vi "(Depricated) AMS Gas.vi"() -> ()   [LabVIEW 2015]
uses:
  Controls/Liquid N Valve Ref Cluster.ctl
  Controls/Main Line Valve Ref Cluster.ctl
  Controls/FP Control Refs Cluster.ctl
  Controls/Sample Valve Refs.ctl
  Controls/AMS Gas State Enumerator.ctl
  Controls/Syringe Ctrl Refs.ctl
  AMS Gas/AMS Gas.lvclass
  <vilib>/ActorFramework/Stop Msg/Stop Msg.lvclass
  AMS Gas Messages/Open Thermocouples Msg/Open Thermocouples Msg.lvclass
  AMS Gas Messages/Open Log Msg/Open Log Msg.lvclass
  Controls/Sample Line State Enumerator.ctl
  AMS Gas Messages/Open Samples Msg/Open Samples Msg.lvclass
  Controls/Sample Transfer Control Enumerator.ctl
  Controls/Sample Push Control Enumerator.ctl
  Controls/Freeze Button.ctl
  Controls/Valve Custom.ctl
  Controls/Sample Transfer Container Enumerator.ctl
  Controls/Sample Transfer State Enumerator.ctl
  Controls/Sample Push State Enumerator.ctl
  Controls/Vacuum State Enumerator.ctl
panel:
  out "Sample Push Progress Slide":u8(slide) scale=0.0..100.0
  out "Sample Transfer Progress Slide":u8(slide) scale=0.0..100.0
  in  "Cylinder Home":bool
  in  "Syringe Blower":bool
  in  "Cylinder Setpoint":dbl=2.6 min=0.0 max=10.0 step=0.01 format="%_3f"
  in  "He Line Valve DV318":bool
  in  "Push Time (sec)":dbl=inf
  out "Vacuum State":T1=enum."Unknown"
  in  "Sample Push Control":T2
  in  "Sample Transfer Control":T3
  out "Sample Push State":T4
  in  "Transfer mBar":dbl min=0.0 step=1.0
  out "cRIO CPU":u8(slide) scale=0.0..100.0
  in  "Transfer Btn":bool
  in  "Target Container":T5
  in  "Source Container":T5
  out "Sample Transfer State":T6
  out "Preparation 1":bool
  out "Capillary 2":bool
  out "Capillary 1":bool
  out "Syringe pipe 1":bool
  out "Syringe pipe 2":bool
  out "Syringe pipe 3":bool
  in  "Monkey Mode":bool
  out "error out":errorcluster
  in  "FV Pump On":bool
  out "Turbo Speed":dbl format="%#_g %"
  in  "Turbo ON":bool
  in  "GV400":bool
  in  "GV401":bool
  out "FV Gauge":dbl format="%^#_3e Pa"
  in  "Open Log":bool
  out "Log":string
  in  "dvPipe 23":bool
  in  "dvPipe 21":bool
  in  "dvPipe 22":bool
  in  "dvPipe 20":bool
  in  "dvPipe 19":bool
  in  "dvPipe 18":bool
  in  "dvPipe 17":bool
  in  "dvPipe 16":bool
  in  "dvPipe 15":bool
  in  "dvPipe 14":bool
  in  "dvPipe 13":bool
  in  "dvPipe 12":bool
  in  "dvPipe 11":bool
  in  "dvPipe 10":bool
  in  "dvPipe 9":bool
  in  "dvPipe 8":bool
  in  "dvPipe 7":bool
  in  "dvPipe 6":bool
  in  "dvPipe 5":bool
  in  "dvPipe 4":bool
  in  "dvPipe 3":bool
  in  "dvPipe 2":bool
  in  "dvPipe 1":bool
  in  "VacLine 2":bool
  in  "VacLine 1":bool
  out "Syringe Position":i32(slide)
  in  "Syringe Setpoint":dbl=1.0 format="%.2f"
  in  "Syringe Enable":bool
  in  "Syringe Run":bool
  in  "Syringe Home":bool
  in  "Syringe Heater":bool
  in  "Piston Heater":bool
  in  "Syringe Freeze":bool
  in  "Syringe TC Graph":bool
  out "Syringe TC":dbl(slide) scale=-200.0..100.0
  out "Syringe Vacuum Gauge PT303":dbl(knob) scale=1.333..1333.0 scale format="%.2e"
  out "Turbo Vacuum Gauge PT302":dbl(knob) scale=1.333..1333.0 scale format="%.2e"
  in  "syrButton":bool
  in  "Liquid N Master Valve HV 107":bool
  in  "Cold Bath Syringe HV 106":bool
  in  "HV315":bool
  in  "HV314":bool
  in  "Turbo Valve DV313":bool
  out "Syringe":dbl(slide) scale=0.0..10.0
  in  "Tank Blower 4":bool
  in  "Tank Blower 3":bool
  in  "Tank Blower 2":bool
  in  "Tank Blower 1":bool
  in  "Cold Bath 1 Freeze":T7
  in  "Cold Bath 2 Freeze":T7
  in  "Cold Bath 3 Freeze":T7
  in  "Cold Bath 4 Freeze":T7
  in  "Clear Charts":bool
  in  "Cold Bath Storage 1 HV 102":T8
  in  "Cold Bath Storage 2 HV 103":T8
  in  "Cold Bath Storage 3 HV 104":bool
  in  "Cold Bath Storage 4 HV 105":bool
  out "Syringe chart":cluster{dbl, dbl}(graph)
  out "TC1":dbl(slide) scale=-200.0..30.0
  out "TC2":dbl(slide) scale=-200.0..30.0
  out "TC3":dbl(slide) scale=-200.0..30.0
  out "TC4":dbl(slide) scale=-200.0..30.0
  out "Baratrons Chart":cluster{"mean":dbl, "mean":dbl}(graph)
  out "Baratron 2":dbl(knob) scale=1.333..1333.0 scale format="%.2e"
  out "Baratron 1":dbl(knob) scale=1.333..1333.0 scale format="%.2e"
  in  "Storage Valve 1":bool
  in  "Prep Line Valve 0 DV300":bool
  in  "Storage Valve 2":bool
  in  "Storage Valve 3":bool
  in  "Storage Valve 4":bool
  in  "Storage Valve 5":bool
  in  "Storage Valve 6":bool
  in  "Storage Valve 7":bool
  in  "Storage Valve 9":bool
  in  "Storage Valve 10":bool
  in  "Storage Valve 11":bool
  in  "Storage Valve 12":bool
  in  "Sample 1 DV314":bool
  in  "Sample 2 DV315":bool
  in  "Sample 3 DV316":bool
  in  "Sample 4 DV317":bool
  in  "Sample 5 DV318":bool
  in  "Storage Valve 8":bool
  in  "Tube 1":bool
  in  "Tube 2":bool
  in  "Tube 3":bool
  in  "Tube 4":bool
  in  "Tube 5":bool
  in  "Tube 6":bool
  in  "Tube 7":bool
  in  "Tube 8":bool
  in  "Tube 9":bool
  in  "Tube 10":bool
  in  "Tube 11":bool
  in  "Tube 12":bool
  in  "Sample 1":bool
  in  "Sample 2":bool
  in  "Sample 3":bool
  in  "Sample 4":bool
  in  "Sample 5":bool
  out "Syringe":bool
  # "VS"
  # "VT"
  # "1"
  # "2"
  # "3"
  # "4"
  # "5"
  # "6"
  # "7"
  # "8"
  # "9"
  # "10"
  # "11"
  # "12"
  # "VIn"
  # "He Line"
  # "1"
  # "2"
  # "3"
  # "4"
  # "5"
  # "Scroll pump"
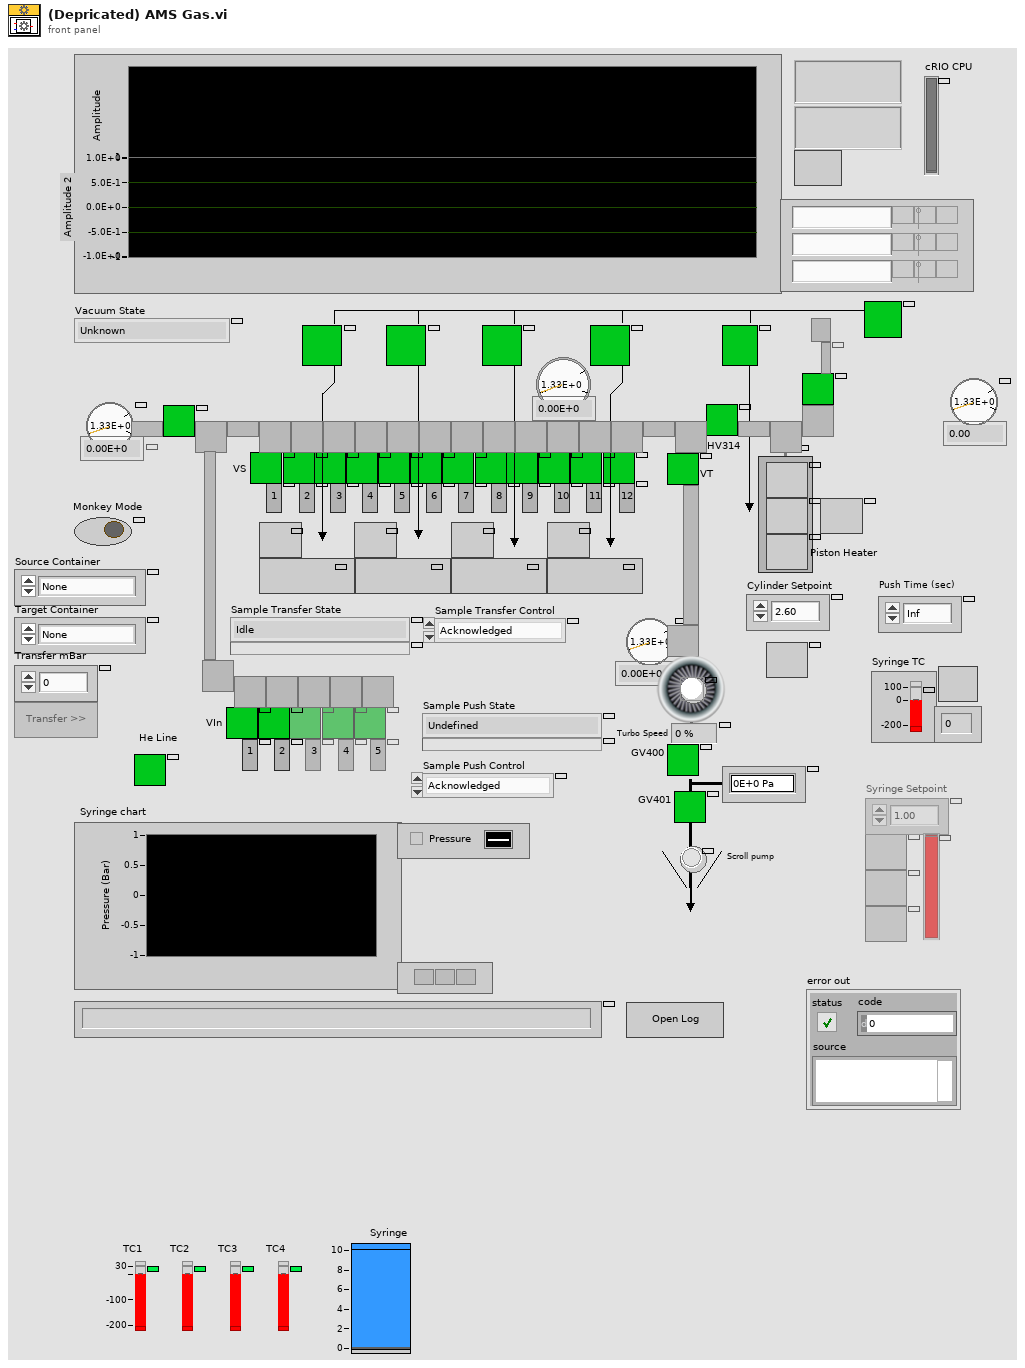
[diagram p1: front panel]
types:
  T1 = typedef "Vacuum State Enumerator.ctl" = enum16{"Pressure Rising", "Plateau", "Pressure Dropping", "Valley", "Low Valley", "Leak", "Unknown"}
  T2 = typedef "Sample Push Control Enumerator.ctl" = enum16{"Acknowledged", "Push", "Stash", "Abort", "Reset to Idle"}
  T3 = typedef "Sample Transfer Control Enumerator.ctl" = enum16{"Acknowledged", "Transfer", "Abort", "Reset to Idle"}
  T4 = typedef "Sample Push State Enumerator.ctl" = enum16{"Undefined", "Initialize", "Dilute", "Close Transfer Line", "Start Heaters", "Warm Up Syringe", "Ready to Push", "Push", "Initiate Stash", "Stash", "Complete", "Abort", "Idle", "Error"}
  T5 = typedef "Sample Transfer Container Enumerator.ctl" = enum16{"None", "Sample 1", "Sample 2", "Sample 3", "Sample 4", "Sample 5", "Storage 01", "Storage 02", "Storage 03", "Storage 04", "Storage 05", "Storage 06", "Storage 07", "Storage 08", "Storage 09", "Storage 10", "Storage 11", "Storage 12", "Syringe", "Undefined"}
  T6 = typedef "Sample Transfer State Enumerator.ctl" = enum16{"Idle", "Initialize", "Check Containers", "Check Temperatures", "Start Turbo", "Warm Up Containers", "Prepare for purging", "Purge Capillary", "Purge", "Open Containers", "Introduce Sample", "Measure Base Pressure", "Home Syringe", "Start Freezer", "Freeze Target", "Crystalize", "Stash", "Polish", "Stop Freezers", "Push Sample", "Complete", "Abort", "Error", "Undefined"}
  T7 = typedef "Freeze Button.ctl" = bool
  T8 = typedef "Valve Custom.ctl" = bool
  T9 = typedef "AMS Gas State Enumerator.ctl" = enum16{"Initialize", "Idle", "Change to Manual", "Change to Auto", "Shutdown"}
  T10 = typedef "FP Control Refs Cluster.ctl" = cluster{"Liquid N Valve References":T11, "Main Line Valve Refs":T12, "Transfer Line Container":refnum<vi>, "Storage Containers":refnum<vi>[], "Sample Refs":T13, "Syringe Ctrl Refs ":T14, "Baratrons Chart":refnum<vi>, "Capillary Container":refnum<vi>, "Preparation Container":refnum<vi>, "Monkey Mode":refnum<vi>}
  T11 = typedef "Liquid N Valve Ref Cluster.ctl" = cluster{"Cold Bath H2O HV 100":refnum<vi>, "Cold Bath Cleaning HV 101":refnum<vi>, "Cold Bath Storage 1 HV 102":refnum<vi>, "Cold Bath Storage 2 HV 103":refnum<vi>, "Cold Bath Storage 3 HV 104":refnum<vi>, "Cold Bath Storage 4 HV 105":refnum<vi>, "Cold Bath Syringe HV 106":refnum<vi>, "Liquid N Master Valve HV 107":refnum<vi>}
  T12 = typedef "Main Line Valve Ref Cluster.ctl" = cluster{"Turbo Valve DV313":refnum<vi>, "Prep Line Valve 0 DV300":refnum<vi>, "Storage Valves":refnum<vi>[]}
  T13 = typedef "Sample Valve Refs.ctl" = cluster{"Valves":cluster{"Sample 5 DV318":refnum<vi>, "Sample 4 DV317":refnum<vi>, "Sample 3 DV316":refnum<vi>, "Sample 2 DV315":refnum<vi>, "Sample 1 DV314":refnum<vi>}, "Lines":cluster{"Sample 1":refnum<vi>, "Sample 2":refnum<vi>, "Sample 3":refnum<vi>, "Sample 4":refnum<vi>, "Sample 5":refnum<vi>}}
  T14 = typedef "Syringe Ctrl Refs.ctl" = cluster{"Syringe Home":refnum<vi>, "Syringe Freeze":refnum<vi>, "Syringe TC":refnum<vi>, "Syringe Container":refnum<vi>}
  T15 = cluster{"Syringe pipe 3":refnum<vi>, "Syringe pipe 2":refnum<vi>, "Syringe pipe 1":refnum<vi>, "Syringe":refnum<vi>}
  T16 = enum8{"Enabled", "Disabled", "Disabled and Grayed Out"}
  T17 = typedef "Sample Line State Enumerator.ctl" = enum16{"All lines closed", "Sample line 1.", "Sample line 2.", "Sample line 3.", "Sample line 4.", "Sample line 5.", "Out of range"}
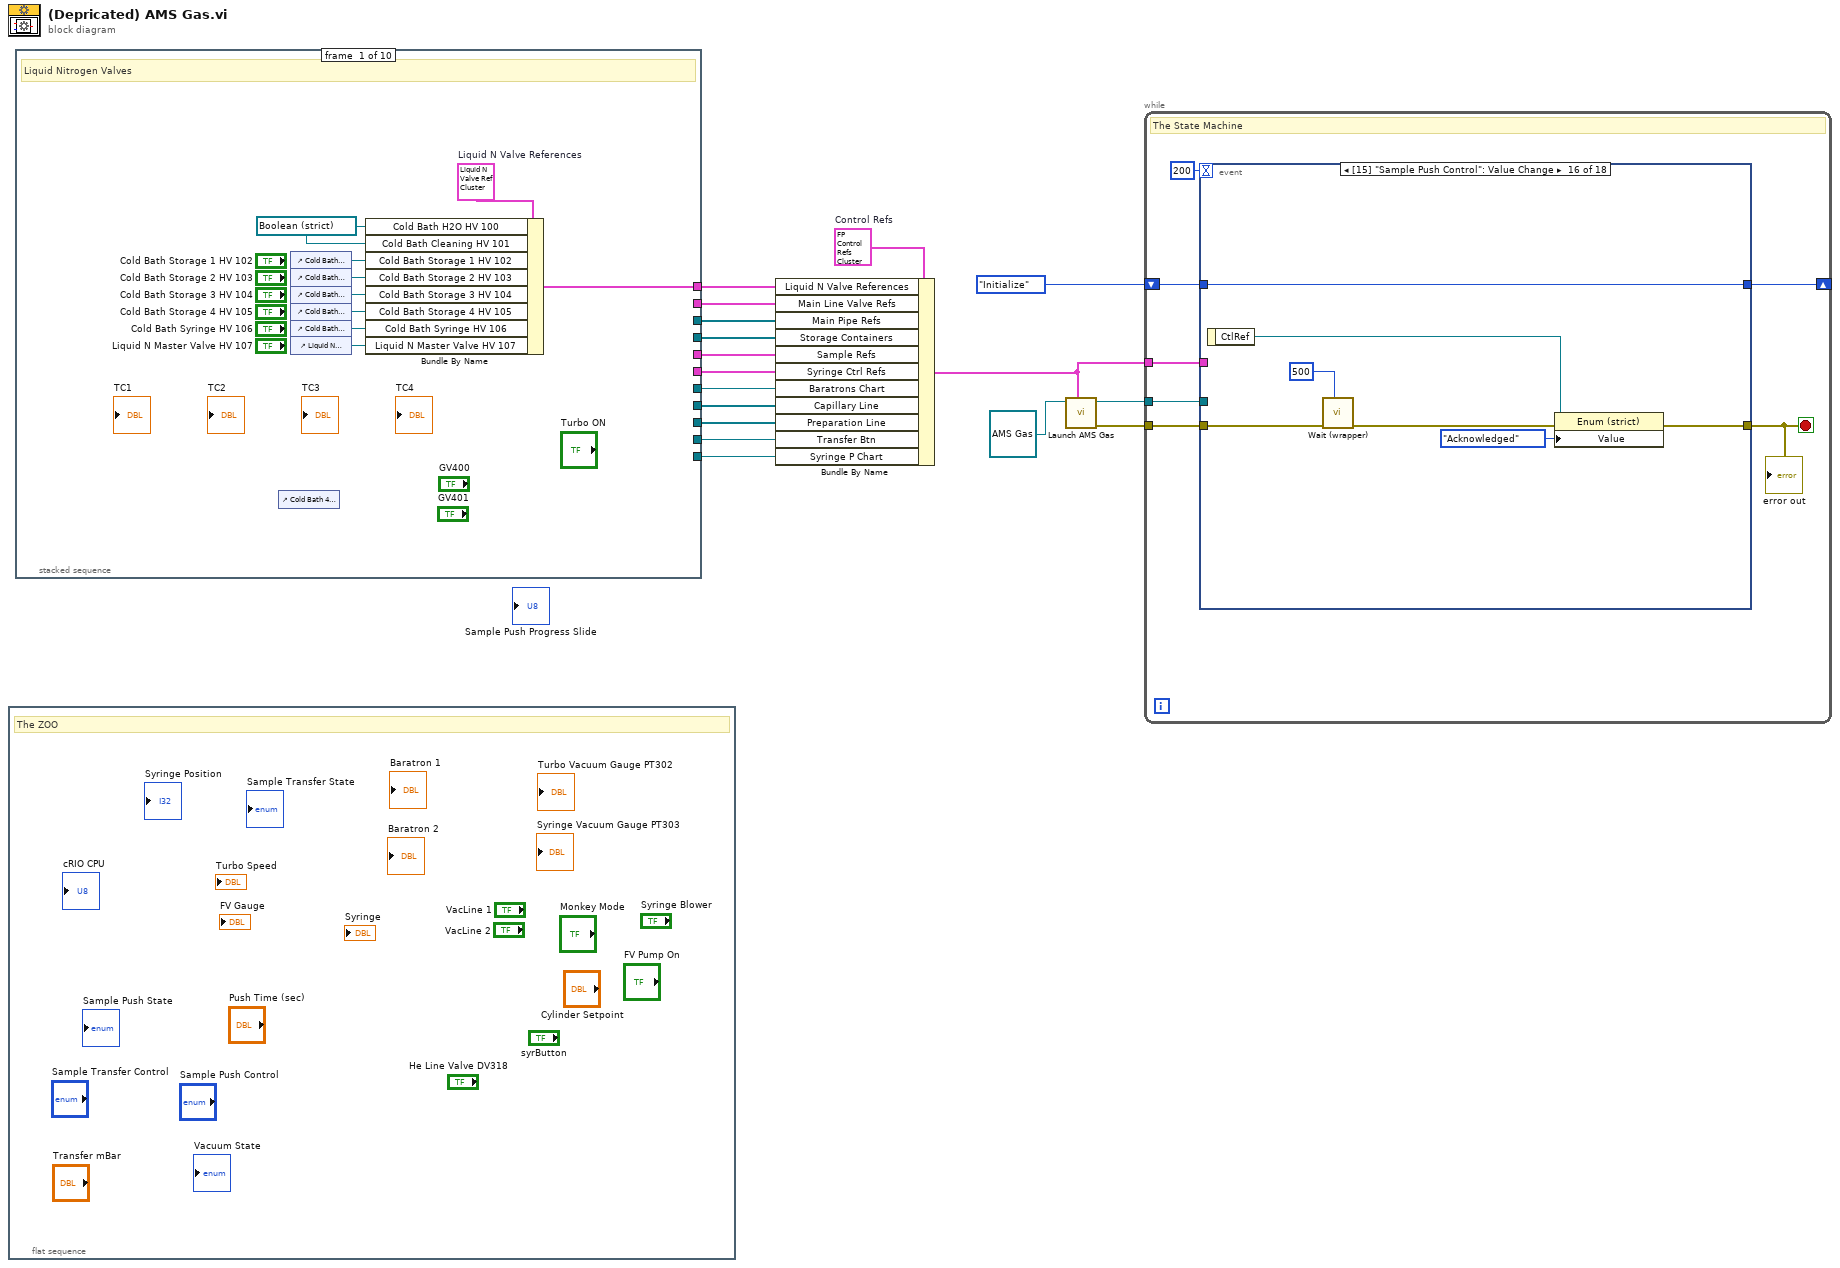
[diagram p0: block diagram]
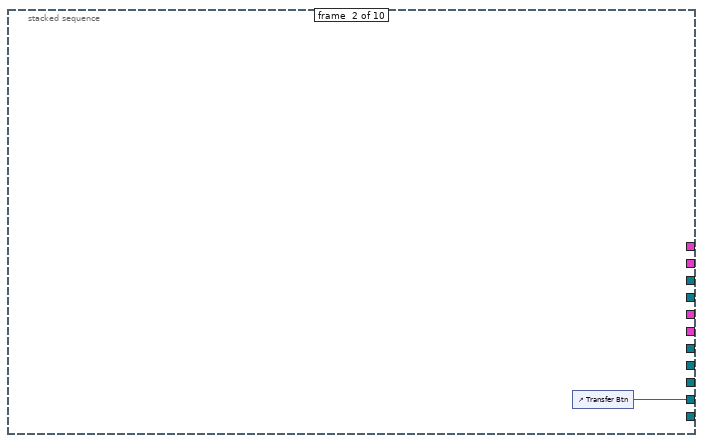
[diagram p2: hidden frame]
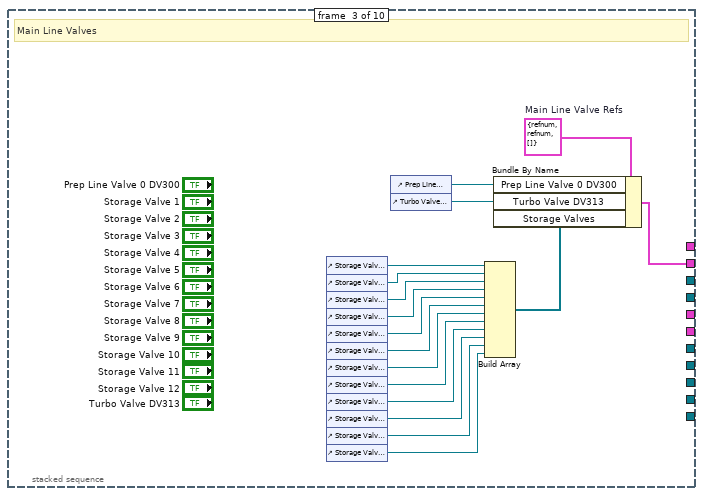
[diagram p3: hidden frame]
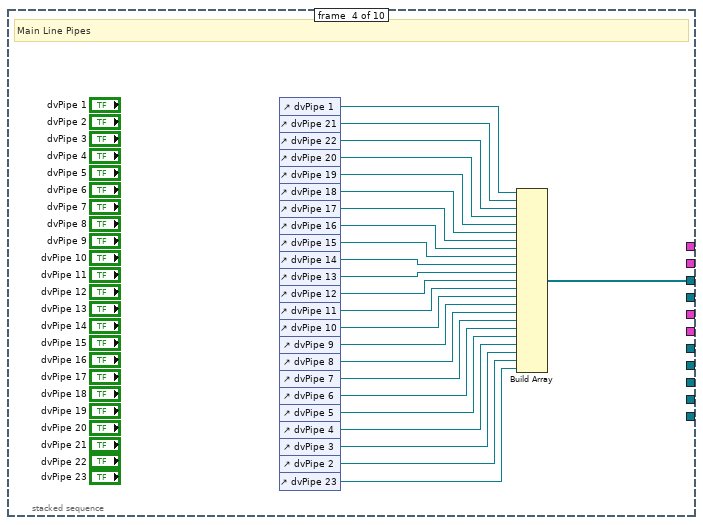
[diagram p4: hidden frame]
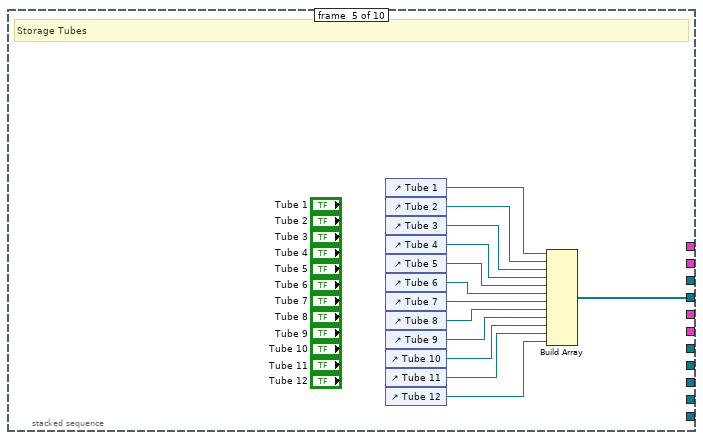
[diagram p5: hidden frame]
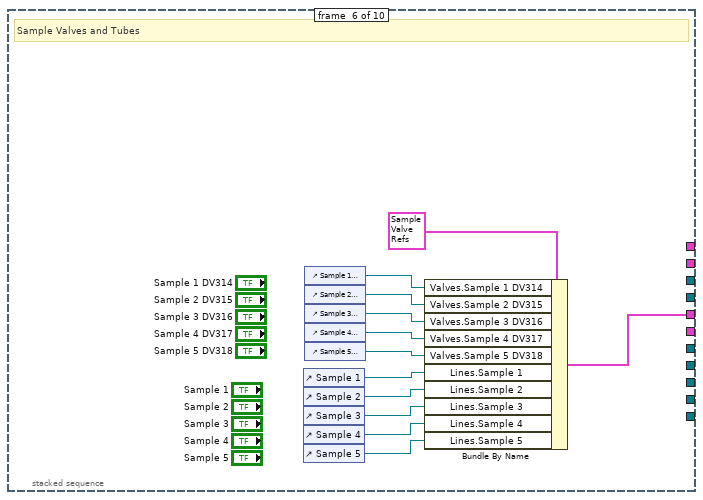
[diagram p6: hidden frame]
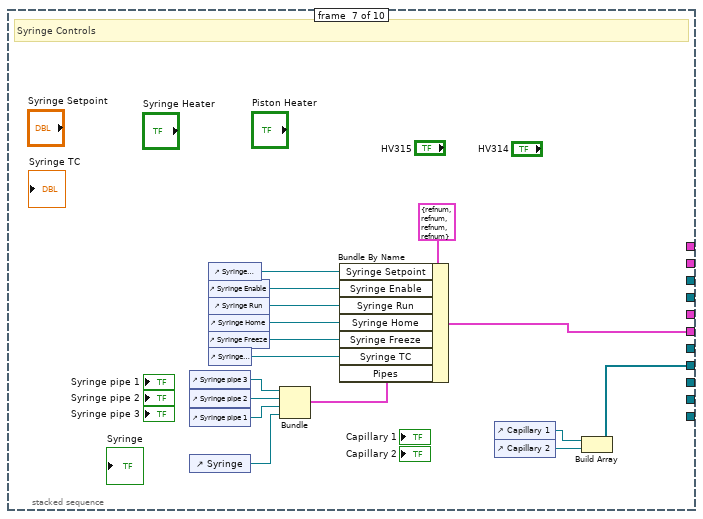
[diagram p7: hidden frame]
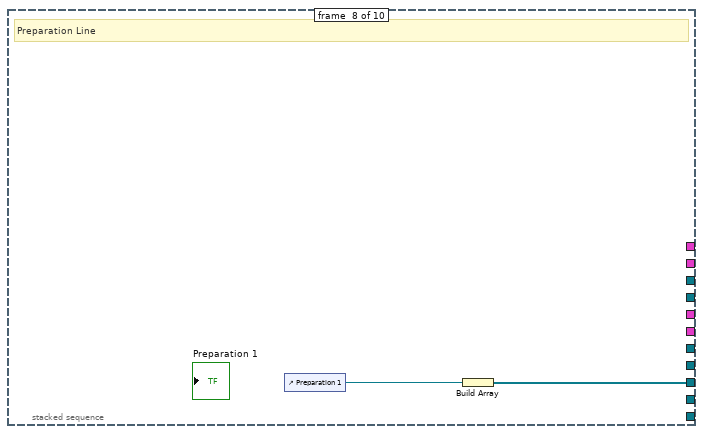
[diagram p8: hidden frame]
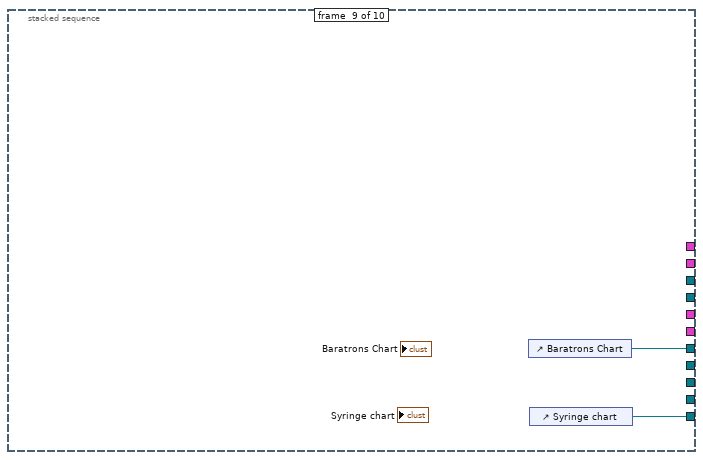
[diagram p9: hidden frame]
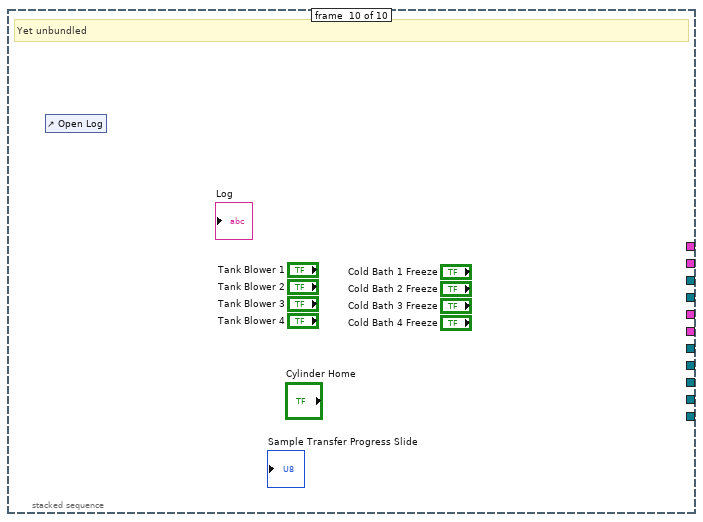
[diagram p10: hidden frame]
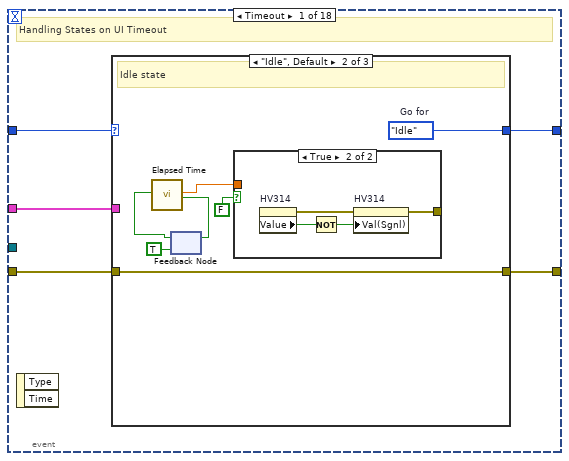
[diagram p11: hidden frame]
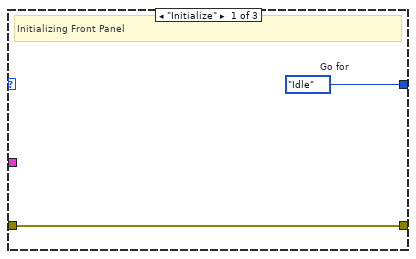
[diagram p12: hidden frame]
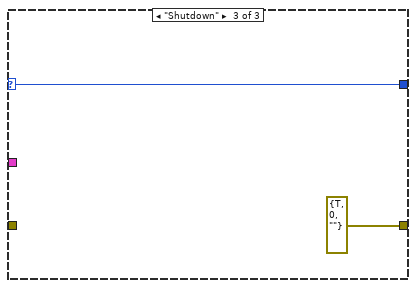
[diagram p14: hidden frame]
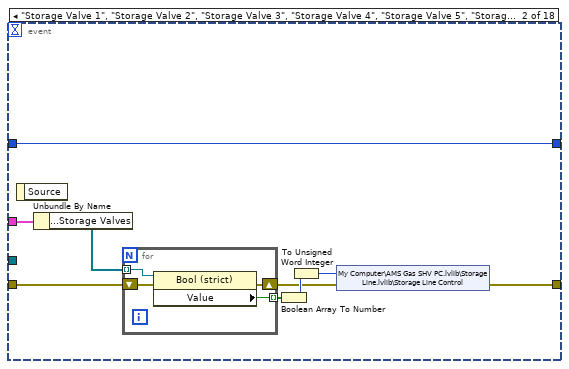
[diagram p15: hidden frame]
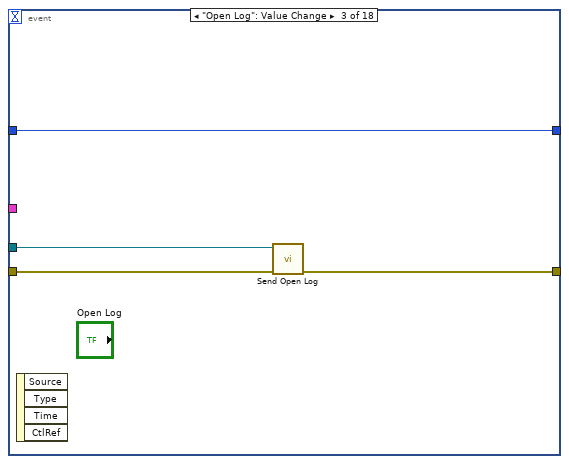
[diagram p16: hidden frame]
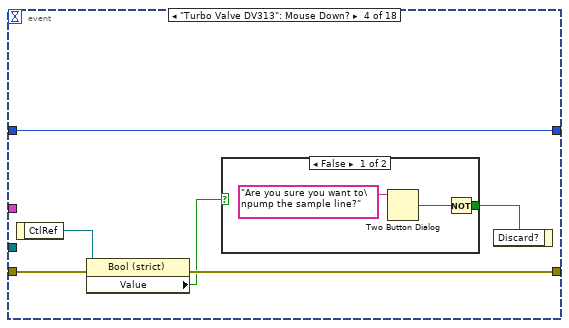
[diagram p17: hidden frame]
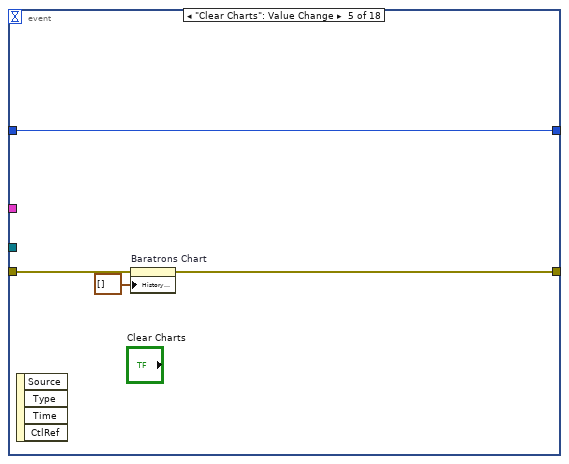
[diagram p19: hidden frame]
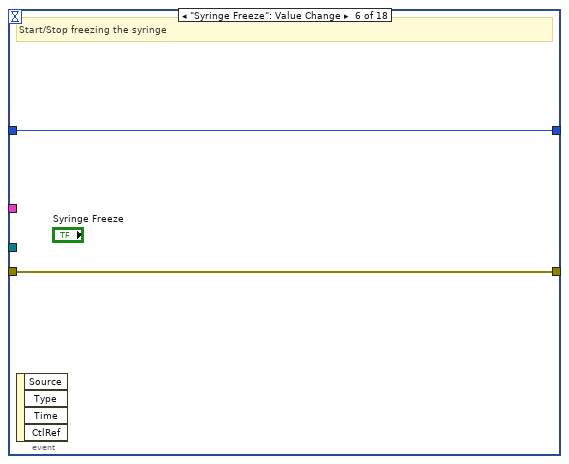
[diagram p20: hidden frame]
diagram:
  w17 = T10 {"Liquid N Valve References"={"Cold Bath H2O HV 100"=refnum, "Cold Bath Cleaning HV 101"=refnum, "Cold Bath Storage 1 HV 102"=refnum, "Cold Bath Storage 2 HV 103"=refnum, "Cold Bath Storage 3 HV 104"=refnum, "Cold Bath Storage 4 HV 105"=refnum, "Cold Bath Syringe HV 106"=refnum, "Liquid N Master Valve HV 107"=refnum}, "Main Line Valve Refs"={"Turbo Valve DV313"=refnum, "Prep Line Valve 0 DV300"=refnum, "Storage Valves"=[]}, "Transfer Line Container"=refnum, "Storage Containers"=[], "Sample Refs"={"Valves"={"Sample 5 DV318"=refnum, "Sample 4 DV317"=refnum, "Sample 3 DV316"=refnum, "Sample 2 DV315"=refnum, "Sample 1 DV314"=refnum}, "Lines"={"Sample 1"=refnum, "Sample 2"=refnum, "Sample 3"=refnum, "Sample 4"=refnum, "Sample 5"=refnum}}, "Syringe Ctrl Refs "={"Syringe Home"=refnum, "Syringe Freeze"=refnum, "Syringe TC"=refnum, "Syringe Container"=refnum}, "Baratrons Chart"=refnum, "Capillary Container"=refnum, "Preparation Container"=refnum, "Monkey Mode"=refnum}  # Control Refs
  n1 = flat-sequence {
    frame #0 {
      # "The ZOO"
    }
  }
  n2 = stacked-sequence {
    tunnel: [_ _ w44 _ _ _ _ _ _ _] -> w16
    tunnel: [_ _ _ w46 _ _ _ _ _ _] -> w14
    tunnel: [_ _ _ _ w69 _ _ _ _ _] -> w12
    tunnel: [_ _ _ _ _ w87 _ _ _ _] -> w11
    tunnel: [w19 _ _ _ _ _ _ _ _ _] -> w13
    tunnel: [_ _ _ _ _ _ w105 _ _ _] -> w10
    tunnel: [_ _ _ _ _ _ _ _ w113 _] -> w7
    tunnel: [_ _ _ _ _ _ w94 _ _ _] -> w5
    tunnel: [_ _ _ _ _ _ _ w110 _ _] -> w4
    tunnel: [_ w27 _ _ _ _ _ _ _ _] -> w3
    tunnel: [_ _ _ _ _ _ _ _ w112 _] -> w1
    frame #0 {
      w18 = refnum<vi> refnum ("Cold Bath H2O HV 100")
      w26 = T11 {"Cold Bath H2O HV 100"=refnum, "Cold Bath Cleaning HV 101"=refnum, "Cold Bath Storage 1 HV 102"=refnum, "Cold Bath Storage 2 HV 103"=refnum, "Cold Bath Storage 3 HV 104"=refnum, "Cold Bath Storage 4 HV 105"=refnum, "Cold Bath Syringe HV 106"=refnum, "Liquid N Master Valve HV 107"=refnum}  # Liquid N Valve References
      # "Liquid Nitrogen Valves"
      n3 = control-ref of="Cold Bath 4 Freeze"() -> ()  [unwired: 1 out]
      n4 = control-ref of="Cold Bath Storage 1 HV 102"() -> (w20:refnum<vi>)
      n5 = control-ref of="Cold Bath Storage 2 HV 103"() -> (w21:refnum<vi>)
      n6 = control-ref of="Cold Bath Storage 3 HV 104"() -> (w22:refnum<vi>)
      n7 = control-ref of="Cold Bath Storage 4 HV 105"() -> (w23:refnum<vi>)
      n8 = control-ref of="Cold Bath Syringe HV 106"() -> (w24:refnum<vi>)
      n9 = control-ref of="Liquid N Master Valve HV 107"() -> (w25:refnum<vi>)
      n10 = Bundle By Name(cluster=w26, "Cold Bath H2O HV 100"=w18, "Cold Bath Cleaning HV 101"=w18, "Cold Bath Storage 1 HV 102"=w20, "Cold Bath Storage 2 HV 103"=w21, "Cold Bath Storage 3 HV 104"=w22, "Cold Bath Storage 4 HV 105"=w23, "Cold Bath Syringe HV 106"=w24, "Liquid N Master Valve HV 107"=w25) -> (w19:T11)
    }
    frame #1 {
      n11 = control-ref of="Transfer Btn"() -> (w27:refnum<vi>)
    }
    frame #2 {
      w42 = T12 {"Turbo Valve DV313"=refnum, "Prep Line Valve 0 DV300"=refnum, "Storage Valves"=[]}  # Main Line Valve Refs
      # "Main Line Valves"
      n12 = control-ref of="Storage Valve 1"() -> (w40:refnum<vi>)
      n13 = control-ref of="Storage Valve 2"() -> (w39:refnum<vi>)
      n14 = control-ref of="Storage Valve 3"() -> (w38:refnum<vi>)
      n15 = control-ref of="Storage Valve 4"() -> (w37:refnum<vi>)
      n16 = control-ref of="Storage Valve 5"() -> (w36:refnum<vi>)
      n17 = control-ref of="Storage Valve 6"() -> (w35:refnum<vi>)
      n18 = control-ref of="Storage Valve 7"() -> (w34:refnum<vi>)
      n19 = control-ref of="Storage Valve 8"() -> (w33:refnum<vi>)
      n20 = control-ref of="Storage Valve 9"() -> (w32:refnum<vi>)
      n21 = control-ref of="Storage Valve 10"() -> (w31:refnum<vi>)
      n22 = control-ref of="Storage Valve 11"() -> (w30:refnum<vi>)
      n23 = control-ref of="Storage Valve 12"() -> (w29:refnum<vi>)
      n24 = control-ref of="Prep Line Valve 0 DV300"() -> (w43:refnum<vi>)
      n25 = control-ref of="Turbo Valve DV313"() -> (w41:refnum<vi>)
      n26 = Build Array(w40, w39, w38, w37, w36, w35, w34, w33, w32, w31, w30, w29) -> (w28:refnum<vi>[])
      n27 = Bundle By Name(cluster=w42, "Prep Line Valve 0 DV300"=w43, "Turbo Valve DV313"=w41, "Storage Valves"=w28) -> (w44:T12)
    }
    frame #3 {
      # "Main Line Pipes"
      n28 = control-ref of="dvPipe 1"() -> (w47:refnum<vi>)
      n29 = control-ref of="dvPipe 21"() -> (w48:refnum<vi>)
      n30 = control-ref of="dvPipe 22"() -> (w49:refnum<vi>)
      n31 = control-ref of="dvPipe 20"() -> (w50:refnum<vi>)
      n32 = control-ref of="dvPipe 19"() -> (w51:refnum<vi>)
      n33 = control-ref of="dvPipe 18"() -> (w52:refnum<vi>)
      n34 = control-ref of="dvPipe 17"() -> (w53:refnum<vi>)
      n35 = control-ref of="dvPipe 16"() -> (w54:refnum<vi>)
      n36 = control-ref of="dvPipe 15"() -> (w55:refnum<vi>)
      n37 = control-ref of="dvPipe 14"() -> (w56:refnum<vi>)
      n38 = control-ref of="dvPipe 13"() -> (w57:refnum<vi>)
      n39 = control-ref of="dvPipe 12"() -> (w58:refnum<vi>)
      n40 = control-ref of="dvPipe 11"() -> (w59:refnum<vi>)
      n41 = control-ref of="dvPipe 10"() -> (w60:refnum<vi>)
      n42 = control-ref of="dvPipe 9"() -> (w61:refnum<vi>)
      n43 = control-ref of="dvPipe 8"() -> (w62:refnum<vi>)
      n44 = control-ref of="dvPipe 7"() -> (w63:refnum<vi>)
      n45 = control-ref of="dvPipe 6"() -> (w64:refnum<vi>)
      n46 = control-ref of="dvPipe 5"() -> (w65:refnum<vi>)
      n47 = control-ref of="dvPipe 4"() -> (w66:refnum<vi>)
      n48 = control-ref of="dvPipe 3"() -> (w67:refnum<vi>)
      n49 = control-ref of="dvPipe 2"() -> (w68:refnum<vi>)
      n50 = control-ref of="dvPipe 23"() -> (w45:refnum<vi>)
      n51 = Build Array(w47, w48, w49, w50, w51, w52, w53, w54, w55, w56, w57, w58, w59, w60, w61, w62, w63, w64, w65, w66, w67, w68, w45) -> (w46:refnum<vi>[])
    }
    frame #4 {
      # "Storage Tubes"
      n52 = control-ref of="Tube 1"() -> (w74:refnum<vi>)
      n53 = control-ref of="Tube 2"() -> (w75:refnum<vi>)
      n54 = control-ref of="Tube 3"() -> (w78:refnum<vi>)
      n55 = control-ref of="Tube 4"() -> (w77:refnum<vi>)
      n56 = control-ref of="Tube 5"() -> (w76:refnum<vi>)
      n57 = control-ref of="Tube 6"() -> (w72:refnum<vi>)
      n58 = control-ref of="Tube 7"() -> (w79:refnum<vi>)
      n59 = control-ref of="Tube 8"() -> (w71:refnum<vi>)
      n60 = control-ref of="Tube 9"() -> (w73:refnum<vi>)
      n61 = control-ref of="Tube 10"() -> (w80:refnum<vi>)
      n62 = control-ref of="Tube 11"() -> (w81:refnum<vi>)
      n63 = control-ref of="Tube 12"() -> (w70:refnum<vi>)
      n64 = Build Array(w74, w75, w78, w77, w76, w72, w79, w71, w73, w80, w81, w70) -> (w69:refnum<vi>[])
    }
    frame #5 {
      # "Sample Valves and Tubes"
      n65 = control-ref of="Sample 1"() -> (w86:refnum<vi>)
      n66 = control-ref of="Sample 2"() -> (w85:refnum<vi>)
      n67 = control-ref of="Sample 3"() -> (w84:refnum<vi>)
      n68 = control-ref of="Sample 4"() -> (w83:refnum<vi>)
      n69 = control-ref of="Sample 5"() -> (w82:refnum<vi>)
      n70 = control-ref of="Sample 1 DV314"() -> (w93:refnum<vi>)
      n71 = control-ref of="Sample 2 DV315"() -> (w92:refnum<vi>)
      n72 = control-ref of="Sample 3 DV316"() -> (w91:refnum<vi>)
      n73 = control-ref of="Sample 4 DV317"() -> (w90:refnum<vi>)
      n74 = control-ref of="Sample 5 DV318"() -> (w89:refnum<vi>)
      n75 = Bundle By Name(cluster=T13 {"Valves"={"Sample 5 DV318"=refnum, "Sample 4 DV317"=refnum, "Sample 3 DV316"=refnum, "Sample 2 DV315"=refnum, "Sample 1 DV314"=refnum}, "Lines"={"Sample 1"=refnum, "Sample 2"=refnum, "Sample 3"=refnum, "Sample 4"=refnum, "Sample 5"=refnum}} ("Sample Valve Refs"), "Valves.Sample 1 DV314"=w93, "Valves.Sample 2 DV315"=w92, "Valves.Sample 3 DV316"=w91, "Valves.Sample 4 DV317"=w90, "Valves.Sample 5 DV318"=w89, "Lines.Sample 1"=w86, "Lines.Sample 2"=w85, "Lines.Sample 3"=w84, "Lines.Sample 4"=w83, "Lines.Sample 5"=w82) -> (w87:T13)
    }
    frame #6 {
      # "Syringe Controls"
      n76 = control-ref of="Syringe pipe 3"() -> (w101:refnum<vi>)
      n77 = control-ref of="Syringe pipe 2"() -> (w100:refnum<vi>)
      n78 = control-ref of="Syringe pipe 1"() -> (w99:refnum<vi>)
      n79 = control-ref of="Syringe"() -> (w97:refnum<vi>)
      n80 = control-ref of="Syringe Setpoint"() -> (w109:refnum<vi>)
      n81 = control-ref of="Syringe Enable"() -> (w108:refnum<vi>)
      n82 = control-ref of="Syringe Run"() -> (w107:refnum<vi>)
      n83 = control-ref of="Syringe Home"() -> (w104:refnum<vi>)
      n84 = control-ref of="Syringe Freeze"() -> (w103:refnum<vi>)
      n85 = control-ref of="Syringe TC"() -> (w102:refnum<vi>)
      n86 = Bundle("Syringe pipe 3"=w101, "Syringe pipe 2"=w100, "Syringe pipe 1"=w99, "Syringe"=w97) -> (w98:T15)  [unwired: 1 in]
      n87 = Bundle By Name(cluster=T14 {"Syringe Home"=refnum, "Syringe Freeze"=refnum, "Syringe TC"=refnum, "Syringe Container"=refnum} ("Syringe Ctrl Refs"), "Syringe Setpoint"=w109, "Syringe Enable"=w108, "Syringe Run"=w107, "Syringe Home"=w104, "Syringe Freeze"=w103, "Syringe TC"=w102, "Pipes"=w98) -> (w105:T14)
      n88 = control-ref of="Capillary 1"() -> (w95:refnum<vi>)
      n89 = control-ref of="Capillary 2"() -> (w96:refnum<vi>)
      n90 = Build Array(w95, w96) -> (w94:refnum<vi>[])
    }
    frame #7 {
      # "Preparation Line"
      n91 = control-ref of="Preparation 1"() -> (w111:refnum<vi>)
      n92 = Build Array(w111) -> (w110:refnum<vi>[])
    }
    frame #8 {
      n93 = control-ref of="Baratrons Chart"() -> (w113:refnum<vi>)
      n94 = control-ref of="Syringe chart"() -> (w112:refnum<vi>)
    }
    frame #9 {
      # "Yet unbundled"
      n95 = control-ref of="Open Log"() -> ()  [unwired: 1 out]
    }
  }
  n96 = Bundle By Name(cluster=w17, "Liquid N Valve References"=w13, "Main Line Valve Refs"=w16, "Main Pipe Refs"=w14, "Storage Containers"=w12, "Sample Refs"=w11, "Syringe Ctrl Refs"=w10, "Baratrons Chart"=w7, "Capillary Line"=w5, "Preparation Line"=w4, "Transfer Btn"=w3, "Syringe P Chart"=w1) -> (w2:T10)
  n97 = call "Launch AMS Gas.vi"("Control Refs"=w2, "AMS Gas in"=refnum<class "AMS Gas.lvclass"> refnum) -> ("error out"=w6:errorcluster, "Caller-To-Actor Enqueuer"=w9:refnum<class "Message Enqueuer.lvclass">)  [unwired: 7 in, 1 out]
  n98 = while {
    tunnel: w2 -> [w115]
    tunnel: w6 -> [w120]
    shift-right: [w116] -> _
    shift-left: AMS_Gas_State_Enumerator."Initialize" ("Go for") -> [w117]
    tunnel: w9 -> [w114]
    stop <- w119 stop-if-true
    # "The State Machine"
    n99 = event shown="[15] \"Sample Push Control\": Value Change" {
      selector: _ -> [_ _ _ _ _ _ _ _ _ _ _ _ _ _ _ _ _ _]
      dyn-events: _ -> [_ _ _ _ _ _ _ _ _ _ _ _ _ _ _ _ _ _]
      timeout: 200 -> [_ _ _ _ _ _ _ _ _ _ _ _ _ _ _ _ _ _]
      tunnel: w120 -> [w125 w147 w156 w161 w170 w171 w173 w177 w181 w195 w199 w233 w244 w246 w253 w295 w303 w314]
      tunnel: [w124 w142 w155 w160 w167 w171 w173 w175 w180 w191 w197 w223 w243 w246 w252 w296 w302 w313] -> w119
      tunnel: w117 -> [w123 w149 w157 w163 w169 w172 w174 w178 _ w187 w202 w234 w245 w247 w256 w299 w301 w312]
      tunnel: [w122 w149 w157 w163 w169 w172 w174 w178 w183 w187 w202 w234 w245 w247 w256 w299 w301 w312] -> w116
      tunnel: w115 -> [w121 w148 _ _ _ _ _ _ _ w196 _ _ _ _ _ _ w304 w315]
      tunnel: w114 -> [_ _ w154 _ _ _ _ w176 w179 _ w201 _ _ _ _ _ _ _]
      event Timeout {
        # "Handling States on UI Timeout"
        n100 = event-data() -> ()  [unwired: 1 in, 2 out]
        n101 = case shown="\"Idle\", Default" w123 {
          selector: w123 -> [_ _ w140]
          tunnel: w125 -> [w126 w133 _]
          tunnel: [w126 w133 errorcluster {"status"=TRUE, "code"=0, "source"=""} ("no error")] -> w124
          tunnel: [w127 w134 w140] -> w122
          tunnel: w121 -> [_ _ _]
          frame "Initialize" {
            w127 = AMS_Gas_State_Enumerator."Idle"  # Go for
            # "Initializing Front Panel"
          }
          frame "Idle", Default {
            w134 = AMS_Gas_State_Enumerator."Idle"  # Go for
            # "Idle state"
            n102 = feedback #1(TRUE ("Time has Elapsed")) -> (w132:bool)
            n103 = call "Elapsed Time"("Reset"=w132) -> ("Elapsed Time (s)"=w130:dbl, "Time has Elapsed"=w129:bool)  [unwired: 11 in, 6 out]
            n104 = feedback-in #1(w129) -> ()
            n105 = case shown="True" FALSE {
              tunnel: [_ w135] -> _
              tunnel: w130 -> [_ _]
              frame False {
              }
              frame True {
                n106 = property on="HV314" class="Bool (strict)"() -> (error out=w136:errorcluster, "Value"=w138:bool)  [unwired: 2 in, 1 out]
                n107 = Not(x=w138) -> (.not. x?=w137:bool)
                n108 = property on="HV314" class="Bool (strict)"(error in=w136, "Val(Sgnl)"=w137) -> (error out=w135:errorcluster)  [unwired: 1 in, 1 out]
              }
            }
          }
          frame "Shutdown" {
          }
        }
      }
      event "Storage Valve 1", "Storage Valve 2", "Storage Valve 3", "Storage Valve 4", "Storage Valve 5", "Storage Valve 6", "Storage Valve 7", "Storage Valve 9", "Storage Valve 10", "Storage Valve 11", "Storage Valve 12", "Storage Valve 8": Value Change {
        n109 = event-data() -> ()  [unwired: 1 in, 1 out]
        n110 = Unbundle By Name(w148) -> ("Main Line Valve Refs.Storage Valves"=w141:refnum<vi>[])
        n111 = for {
          tunnel: w141 -> [w151] mode=indexing
          tunnel: [w150] -> w146 mode=indexing
          shift-right: [w152] -> w144
          shift-left: w147 -> [w153]
          n112 = property class="Bool (strict)"(reference=w151, error in=w153) -> (error out=w152:errorcluster, "Value"=w150:bool)  [unwired: 1 out]
        }
        n113 = Boolean Array To Number(Boolean array=w146) -> (number=w145:u32)
        n114 = To Unsigned Word Integer(number=w145) -> (unsigned 16bit integer=w143:u16)
        n115 = shared-variable "My Computer\\AMS Gas SHV PC.lvlib\\Storage Line.lvlib\\Storage Line Control"(w143, error in=w144) -> (error out=w142:errorcluster)
      }
      event "Open Log": Value Change {
        n116 = event-data() -> ()  [unwired: 1 in, 4 out]
        n117 = call "Send Open Log.vi"("error in (no error)"=w156, "Message Enqueuer"=w154) -> ("error out"=w155:errorcluster)  [unwired: 8 in, 1 out]
      }
      event "Turbo Valve DV313": Mouse Down? {
        n118 = event-data() -> ("CtlRef"=w159:refnum<vi>)  [unwired: 1 in]
        n119 = property class="Bool (strict)"(reference=w159, error in=w161) -> (error out=w160:errorcluster, "Value"=w158:bool)  [unwired: 1 out]
        n120 = case shown="False" w158 {
          tunnel: [w165 _] -> w162
          frame False {
            n121 = Two Button Dialog(message="Are you sure you want to\npump the sample line?") -> (T button?=w166:bool)  [unwired: 2 in]
            n122 = Not(x=w166) -> (.not. x?=w165:bool)
          }
          frame True {
          }
        }
        n123 = event-data("Discard?"=w162) -> ()  [unwired: 1 in, 1 out]
      }
      event "Clear Charts": Value Change {
        n124 = event-data() -> ()  [unwired: 1 in, 4 out]
        n125 = property on="Baratrons Chart" class="WFChart (strict)"(error in=w170, "History Data"=cluster{"mean":dbl, "mean":dbl}[] []) -> (error out=w167:errorcluster)  [unwired: 1 in, 1 out]
      }
      event "Syringe Freeze": Value Change {
        # "Start/Stop freezing the syringe"
        n126 = event-data() -> ()  [unwired: 1 in, 4 out]
      }
      event Value Change {
        # "Start/Stop freezing the Cold Bath 4"
        n127 = event-data() -> ()  [unwired: 1 in, 4 out]
      }
      event "Syringe TC Graph": Value Change {
        n128 = event-data() -> ()  [unwired: 1 in, 4 out]
        n129 = call "Send Open Thermocouples.vi"("error in (no error)"=w177, "Message Enqueuer"=w176) -> ("error out"=w175:errorcluster)  [unwired: 8 in, 1 out]
      }
      event Panel Close? {
        w183 = AMS_Gas_State_Enumerator."Shutdown"  # Go for
        # "User closes Front Panel"
        n130 = event-data() -> ()  [unwired: 1 in, 3 out]
        n131 = call <vilib>:"Send Normal Stop.vi"("error in (no error)"=w181, "Message Enqueuer"=w179) -> ("error out"=w180:errorcluster)  [unwired: 9 in]
        n132 = event-data("Discard?"=TRUE) -> ()  [unwired: 1 in, 1 out]
      }
      event "Syringe Enable": Value Change {
        n133 = event-data() -> ()  [unwired: 1 in, 4 out]
        n134 = Unbundle By Name(w196) -> ("Syringe Run"=w192:refnum<vi>, "Syringe Ctrl Refs.Syringe Home"=w193:refnum<vi>)
        n135 = Select(t=T16."Enabled" ("Disabled"), s="Syringe Enable", f=T16."Disabled and Grayed Out" ("Disabled")) -> (s? t:f=w186:T16)
        n136 = property class="Bool (strict)"(reference=w193, error in=w195, "Value"=FALSE, "DisabledEnum"=w186) -> (error out=w194:errorcluster)  [unwired: 1 out]
        n137 = property class="Bool (strict)"(reference=w192, error in=w194, "Value"=FALSE, "DisabledEnum"=w186) -> (error out=w191:errorcluster)  [unwired: 1 out]
      }
      event "Sample 1", "Sample 2", "Sample 3", "Sample 4", "Sample 5": Mouse Down? {
        n138 = event-data() -> ("CtlRef"=w198:refnum<vi>)  [unwired: 1 in]
        n139 = disable-structure shown="Disabled" {
          disable-tunnel: w201 -> [w211 w220]
          disable-tunnel: w199 -> [w210 w222]
          disable-tunnel: w198 -> [w208 _]
          disable-tunnel: [w205 w221] -> w197
          frame Disabled {
            n140 = property class="Bool (strict)"(reference=w208, error in=w210) -> (reference out=w203:refnum<vi>, error out=w209:errorcluster, "Label.Text"=w204:string)
            n141 = call "(Depricated) Dialog Sample.vi"("Sample Line Control Ref"=w203, "Error In"=w209, "Caller-To-Actor Enqueuer"=w211) -> ("Error Out"=w207:errorcluster, "Sample Removed"=w206:bool)  [unwired: 6 in, 1 out]
            n142 = case shown="False" w206 {
              tunnel: w207 -> [w212 w214]
              tunnel: [w212 w213] -> w205
              tunnel: w204 -> [_ w215]
              frame False {
              }
              frame True {
                n143 = case shown="\"Sample 1\"" w215 {
                  tunnel: w214 -> [w218 w219]
                  tunnel: [w217 w219] -> w213
                  frame "Sample 1" {
                    n144 = shared-variable "My Computer\\AMS Gas SHV PC.lvlib\\Valves.lvlib\\Sample Line Valves.lvlib\\Sample Line 1"(FALSE ("Sample Line 1"), error in=w218) -> (error out=w217:errorcluster)
                  }
                  frame "True", Default {
                  }
                }
              }
            }
          }
          frame Enabled {
            n145 = call "Send Open Samples.vi"("error in (no error)"=w222, "Message Enqueuer"=w220) -> ("error out"=w221:errorcluster)  [unwired: 8 in, 1 out]
          }
        }
        n146 = event-data("Discard?"=TRUE) -> ()  [unwired: 1 in, 1 out]
      }
      event "Sample 1 DV314", "Sample 2 DV315", "Sample 3 DV316", "Sample 4 DV317", "Sample 5 DV318": Mouse Down? {
        n147 = event-data() -> ("CtlRef"=w232:refnum<vi>)  [unwired: 1 in, 1 out]
        n148 = property class="Bool (strict)"(reference=w232, error in=w233) -> (error out=w224:errorcluster, "Label.Text"=w230:string, "Value"=w229:bool)  [unwired: 1 out]
        n149 = Not(x=w229) -> (.not. x?=w228:bool)
        n150 = case shown="\"Sample 2 DV315\"" w230 {
          tunnel: [Sample_Line_State_Enumerator."All lines closed" ("Sample Line") Sample_Line_State_Enumerator."Sample line 1." ("Sample Line") Sample_Line_State_Enumerator."Sample line 2." ("Sample Line")] -> w227
          frame "False", Default {
          }
          frame "Sample 1 DV314" {
          }
          frame "Sample 2 DV315" {
          }
        }
        n151 = Select(t=w227, s=w228, f=Sample_Line_State_Enumerator."All lines closed") -> (s? t:f=w225:T17)
        n152 = shared-variable "My Computer\\AMS Gas SHV PC.lvlib\\Sample Lines.lvlib\\Sample Line Control"(w225, error in=w224) -> (error out=w223:errorcluster)
        n153 = event-data("Discard?"=TRUE) -> ()  [unwired: 1 in, 1 out]
      }
      event "Transfer Btn": Value Change {
        n154 = event-data() -> ()  [unwired: 1 in, 6 out]
        n155 = Select(t=Sample_Transfer_Control_Enumerator."Transfer" ("Sample Transfer Control"), s="Transfer Btn", f=Sample_Transfer_Control_Enumerator."Abort") -> (s? t:f=w238:T3)
        n156 = shared-variable-write(refnum<k21> "ni.var.psp://localhost/AMS Gas SHV PC/Sample Transfer/Control" ("shared variable refnum in"), w244, w238) -> (w243:errorcluster)  [unwired: 1 out]
      }
      event "Tube 1", "Tube 2", "Tube 3", "Tube 4", "Tube 5", "Tube 6", "Tube 7", "Tube 9", "Tube 10", "Tube 11", "Tube 12": Mouse Down {
        n157 = event-data() -> ()  [unwired: 1 in, 1 out]
      }
      event Value Change {
        n158 = event-data() -> ()  [unwired: 1 in, 6 out]
        n159 = case shown="\"Storage 04\"..\"Storage 06\"" "Source Container" {
          tunnel: [w258 w263 w269 w275 w281 w287 FALSE] -> _
          tunnel: "Target Container" -> [w257 w262 w268 w274 w280 w286 _]
          frame "Sample 1".."Sample 5" {
            n160 = case shown="\"Storage 01\", Default" w257 {
              tunnel: [TRUE FALSE FALSE] -> w258
              frame "Storage 01", Default {
              }
              frame "Sample 1".."Sample 5" {
              }
              frame "Undefined" {
              }
            }
          }
          frame "Storage 01".."Storage 03" {
            n161 = case shown="\"Storage 04\"..\"Syringe\"" w262 {
              tunnel: [TRUE FALSE FALSE FALSE] -> w263
              frame "Storage 04".."Syringe" {
              }
              frame "Storage 01".."Storage 03" {
              }
              frame "Sample 1".."Sample 5" {
              }
              frame "Undefined", Default {
              }
            }
          }
          frame "Storage 04".."Storage 06" {
            n162 = case shown="\"Undefined\", Default" w268 {
              tunnel: [TRUE FALSE FALSE FALSE] -> w269
              frame "Storage 01".."Storage 03", "Storage 07".."Syringe" {
              }
              frame "Storage 04".."Storage 06" {
              }
              frame "Sample 1".."Sample 5" {
              }
              frame "Undefined", Default {
              }
            }
          }
          frame "Storage 07".."Storage 09" {
            n163 = case shown="\"Sample 1\"..\"Sample 5\"" w274 {
              tunnel: [TRUE FALSE FALSE FALSE] -> w275
              frame "Storage 01".."Storage 06", "Storage 10".."Syringe" {
              }
              frame "Storage 07".."Storage 09" {
              }
              frame "Sample 1".."Sample 5" {
              }
              frame "Undefined", Default {
              }
            }
          }
          frame "Storage 10".."Storage 12" {
            n164 = case shown="\"Undefined\", Default" w280 {
              tunnel: [TRUE FALSE FALSE FALSE] -> w281
              frame "Storage 01".."Storage 09", "Syringe" {
              }
              frame "Storage 10".."Storage 12" {
              }
              frame "Sample 1".."Sample 5" {
              }
              frame "Undefined", Default {
              }
            }
          }
          frame "Syringe" {
            n165 = case shown="\"Sample 1\"..\"Sample 5\"" w286 {
              tunnel: [TRUE FALSE FALSE FALSE] -> w287
              frame "Storage 01".."Storage 12" {
              }
              frame "Sample 1".."Sample 5" {
              }
              frame "Syringe" {
              }
              frame "Undefined", Default {
              }
            }
          }
          frame "Undefined", Default {
          }
        }
        n166 = Select(t=T16."Enabled" ("Disabled"), s=FALSE, f=T16."Disabled and Grayed Out") -> (s? t:f=w251:T16)
        n167 = property on="Transfer Btn" class="Bool (strict)"(error in=w253, "DisabledEnum"=w251) -> (error out=w252:errorcluster)  [unwired: 1 in, 1 out]
      }
      event Value Change {
        n168 = event-data() -> ("CtlRef"=w298:refnum<vi>)  [unwired: 1 in]
        n169 = call "Wait (wrapper).vi"("milliseconds to wait (200)"=u32 500, "error in (no error)"=w295) -> ("error out"=w294:errorcluster)  [unwired: 9 in]
        n170 = property class="Enum (strict)"(reference=w298, error in=w294, "Value"=Sample_Push_Control_Enumerator."Acknowledged") -> (error out=w296:errorcluster)  [unwired: 1 out]
      }
      event "Syringe Home": Value Change {
        n171 = event-data() -> ()  [unwired: 1 in, 4 out]
        n172 = case shown="True" "Syringe Home" {
          tunnel: w304 -> [_ w310]
          tunnel: w303 -> [w305 w309]
          tunnel: [w305 w307] -> w302
          frame False {
          }
          frame True {
            n173 = Unbundle By Name(w310) -> ("Syringe Run"=w308:refnum<vi>)
            n174 = property class="Bool (strict)"(reference=w308, error in=w309, "Value"=FALSE) -> (error out=w307:errorcluster)  [unwired: 1 out]
          }
        }
      }
      event "Syringe Run": Value Change {
        n175 = event-data() -> ()  [unwired: 1 in, 4 out]
        n176 = case shown="True" "Syringe Run" {
          tunnel: w315 -> [_ w321]
          tunnel: w314 -> [w316 w320]
          tunnel: [w316 w318] -> w313
          frame False {
          }
          frame True {
            n177 = Unbundle By Name(w321) -> ("Syringe Ctrl Refs.Syringe Home"=w319:refnum<vi>)
            n178 = property class="Bool (strict)"(reference=w319, error in=w320, "Value"=FALSE) -> (error out=w318:errorcluster)  [unwired: 1 out]
          }
        }
      }
    }
    "error out" <- w119
  }
